vi "Read configuration.vi"(8 "error in (no error)":errorcluster, 11 "Digitizer Channel":refnum<class "Digitizer Channel.lvclass">) -> (0 "error out":errorcluster, 2 "configuration":refnum<class "CEF_serializable configuration.lvclass">, 3 "Digitizer Channel out":refnum<class "Digitizer Channel.lvclass">)   [LabVIEW 2025, in "Digitizer.lvlib" / "Digitizer Channel.lvclass"]
uses:
  Digitizer Channel.lvclass
  Users/Public/Documents/Sandia National Labs/TSS Plugin/CEF.lvlibp/serializable configuration/CEF_serializable configuration.lvclass
  Digitizer Channel.lvclass/Digitizer Channel.ctl
  Digitizer Channel configuration/Digitizer Channel configuration.lvclass
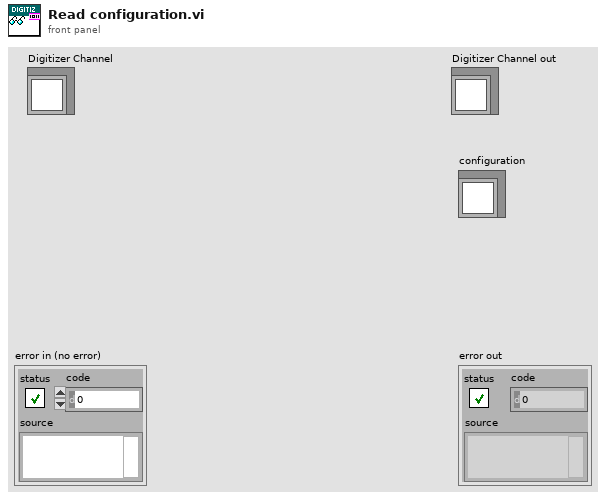
[diagram p1: front panel]
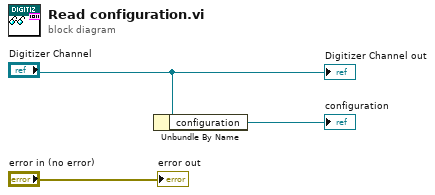
[diagram p0: block diagram]
diagram:
  n1 = Unbundle By Name("Digitizer Channel") -> ("configuration"=→"configuration":refnum<class "Digitizer Channel configuration.lvclass">)
  "error out" <- "error in (no error)"
  "Digitizer Channel out" <- "Digitizer Channel"
